vi "niDTS WLAN UTIL Type to OFDM Rate.vi"(10 "WLAN Type":T2) -> (2 "OFDM Data Rate (Mbps)":T1)   [LabVIEW 2015, in "niDTS WLAN.lvlib"]
uses:
  niDTS WLAN.lvlib
  Includes/niDTS WLAN INC Type.ctl
  Includes/niDTS WLAN INC OFDM Data Rate.ctl
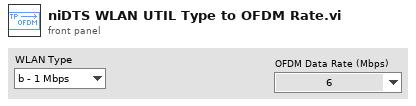
[diagram p1: front panel]
types:
  T1 = typedef "niDTS WLAN.lvlib/niDTS WLAN INC OFDM Data Rate.ctl" = enum16{"6", "9", "12", "18", "24", "36", "48", "54"}
  T2 = typedef "niDTS WLAN.lvlib/niDTS WLAN INC Type.ctl" = enum16{"b - 1 Mbps", "b - 2 Mbps", "b - 5.5 Mbps", "b - 11 Mbps", "ag - 6 Mbps", "ag - 9 Mbps", "ag - 12 Mbps", "ag - 18 Mbps", "ag - 24 Mbps", "ag - 36 Mbps", "ag - 48 Mbps", "ag - 54 Mbps", "n - MCS0", "n - MCS1", "n - MCS2", "n - MCS3", "n - MCS4", "n - MCS5", "n - MCS6", "n - MCS7", "n - MCS8", "n - MCS9", "n - MCS10", "n - MCS11", "n - MCS12", "n - MCS13", "n - MCS14", "n - MCS15", "n - MCS16", "n - MCS17", "n - MCS18", "n - MCS19", "n - MCS20", "n - MCS21", "n - MCS22", "n - MCS23", "n - MCS24", "n - MCS25", "n - MCS26", "n - MCS27", "n - MCS28", "n - MCS29", "n - MCS30", "n - MCS31", "ac - MCS0 -1", "ac - MCS1 -1", "ac - MCS2 -1", "ac - MCS3 -1", "ac - MCS4 -1", "ac - MCS5 -1", "ac - MCS6 -1", "ac - MCS7 -1", "ac - MCS8 -1", "ac - MCS9 -1", "ac - MCS0 -2", "ac - MCS1 -2", "ac - MCS2 -2", "ac - MCS3 -2", "ac - MCS4 -2", "ac - MCS5 -2", "ac - MCS6 -2", "ac - MCS7 -2", "ac - MCS8 -2", "ac - MCS9 -2", "ac - MCS0 -3", "ac - MCS1 -3", "ac - MCS2 -3", "ac - MCS3 -3", "ac - MCS4 -3", "ac - MCS5 -3", "ac - MCS6 -3", "ac - MCS7 -3", "ac - MCS8 -3", "ac - MCS9 -3", "ac - MCS0 -4", "ac - MCS1 -4", "ac - MCS2 -4", "ac - MCS3 -4", "ac - MCS4 -4", "ac - MCS5 -4", "ac - MCS6 -4", "ac - MCS7 -4", "ac - MCS8 -4", "ac - MCS9 -4"}
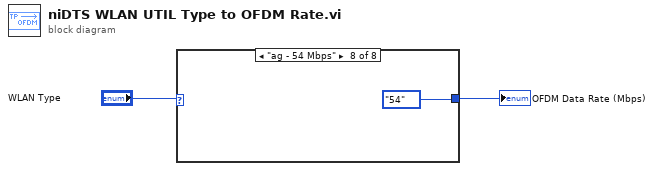
[diagram p0: block diagram]
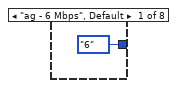
[diagram p2: hidden frame]
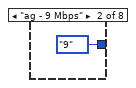
[diagram p3: hidden frame]
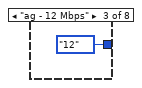
[diagram p4: hidden frame]
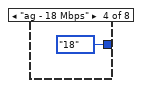
[diagram p5: hidden frame]
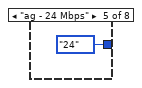
[diagram p6: hidden frame]
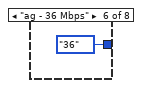
[diagram p7: hidden frame]
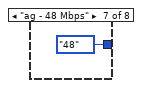
[diagram p8: hidden frame]
diagram:
  n1 = case shown="\"ag - 54 Mbps\"" "WLAN Type" {
    tunnel: [niDTS_WLAN_INC_OFDM_Data_Rate."6" ("OFDM Data Rate (Mbps)") niDTS_WLAN_INC_OFDM_Data_Rate."9" ("OFDM Data Rate (Mbps)") niDTS_WLAN_INC_OFDM_Data_Rate."12" ("OFDM Data Rate (Mbps)") niDTS_WLAN_INC_OFDM_Data_Rate."18" ("OFDM Data Rate (Mbps)") niDTS_WLAN_INC_OFDM_Data_Rate."24" ("OFDM Data Rate (Mbps)") niDTS_WLAN_INC_OFDM_Data_Rate."36" ("OFDM Data Rate (Mbps)") niDTS_WLAN_INC_OFDM_Data_Rate."48" ("OFDM Data Rate (Mbps)") niDTS_WLAN_INC_OFDM_Data_Rate."54" ("OFDM Data Rate (Mbps)")] -> w1
    frame "ag - 6 Mbps", Default {
    }
    frame "ag - 9 Mbps" {
    }
    frame "ag - 12 Mbps" {
    }
    frame "ag - 18 Mbps" {
    }
    frame "ag - 24 Mbps" {
    }
    frame "ag - 36 Mbps" {
    }
    frame "ag - 48 Mbps" {
    }
    frame "ag - 54 Mbps" {
    }
  }
  "OFDM Data Rate (Mbps)" <- w1
